vi "PRT1_Vi.vi"() -> ()   [LabVIEW 2020]
uses:
  <vilib>/Analysis/3filter.llb/Filter Passband Type.ctl
  <vilib>/Analysis/3filter.llb/Butterworth Filter (DBL).vi
  <vilib>/Analysis/NI_AALBase.lvlib
  <vilib>/ptbypt/NI_PtbyPt.lvlib
panel:
  out "FLUX_GRAPH":dbl(graph)
  out "VOLUME_GRAPH":dbl(graph)
  out "VOLUME [ L ]":dbl
  out "VOLUME_TANK [L]":dbl(slide) scale=0.0..4.0
  out "UPDATED":bool
  out "Respiratoy Rate [bpm]":dbl format="%#_3g"
  out "RESPIRATORY COUNT":dbl
  out "SYSTEM OK":bool
  out "MEAN ERROR":dbl format="%#_4g"
  out "INSPIRATION":bool
  out "SPIRATION":bool
  out "FILTERED VOLTAGE [V]":dbl
  out "VOLTAGE":dbl[](graph)
  in  "STOP SYSTEM":bool
  out "PRESSURE CHART":dbl(graph)
  out "FLUX [L/m]":dbl format="%#_4g"
  out "SPEED[cm/s]":dbl format="%#_4g"
  out "PRESSURE":dbl format="%#_4g"
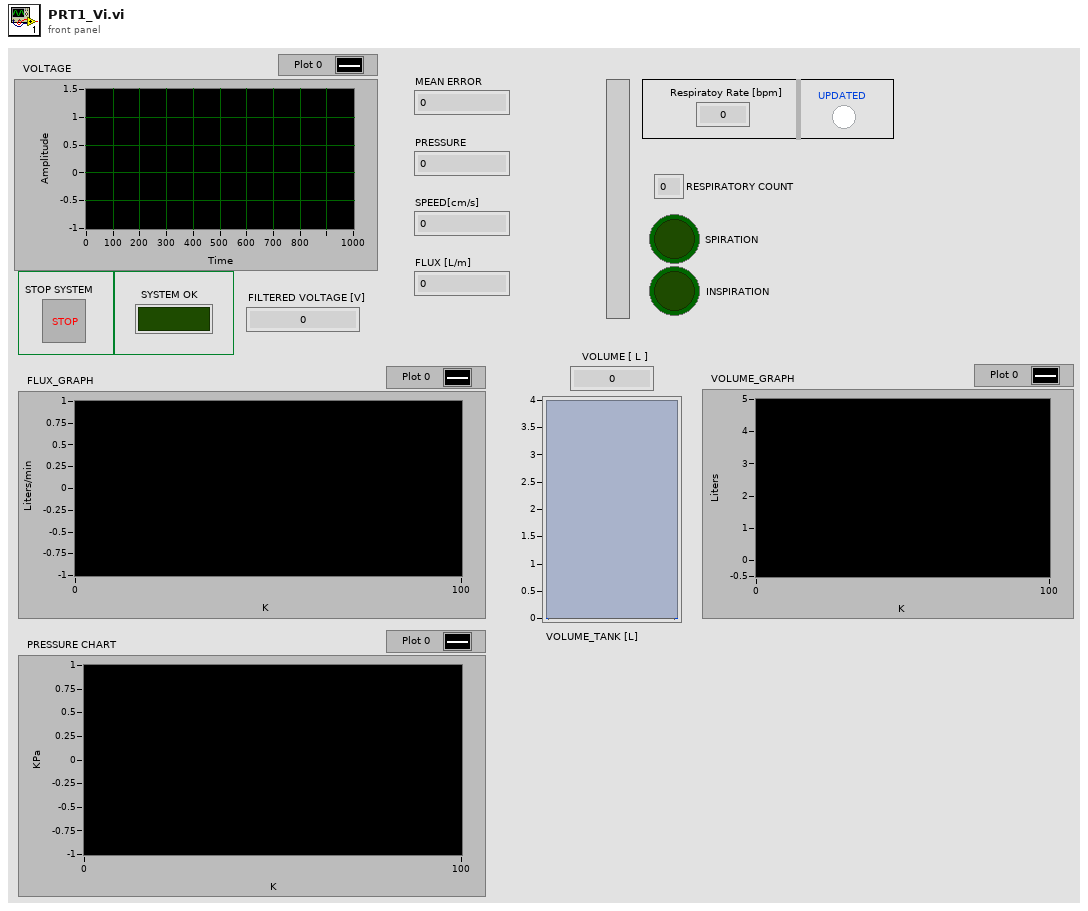
[diagram p1: front panel]
types:
  T1 = typedef "NI_AALBase.lvlib/Filter Passband Type.ctl" = enum32{"Lowpass", "Highpass", "Bandpass", "Bandstop"}
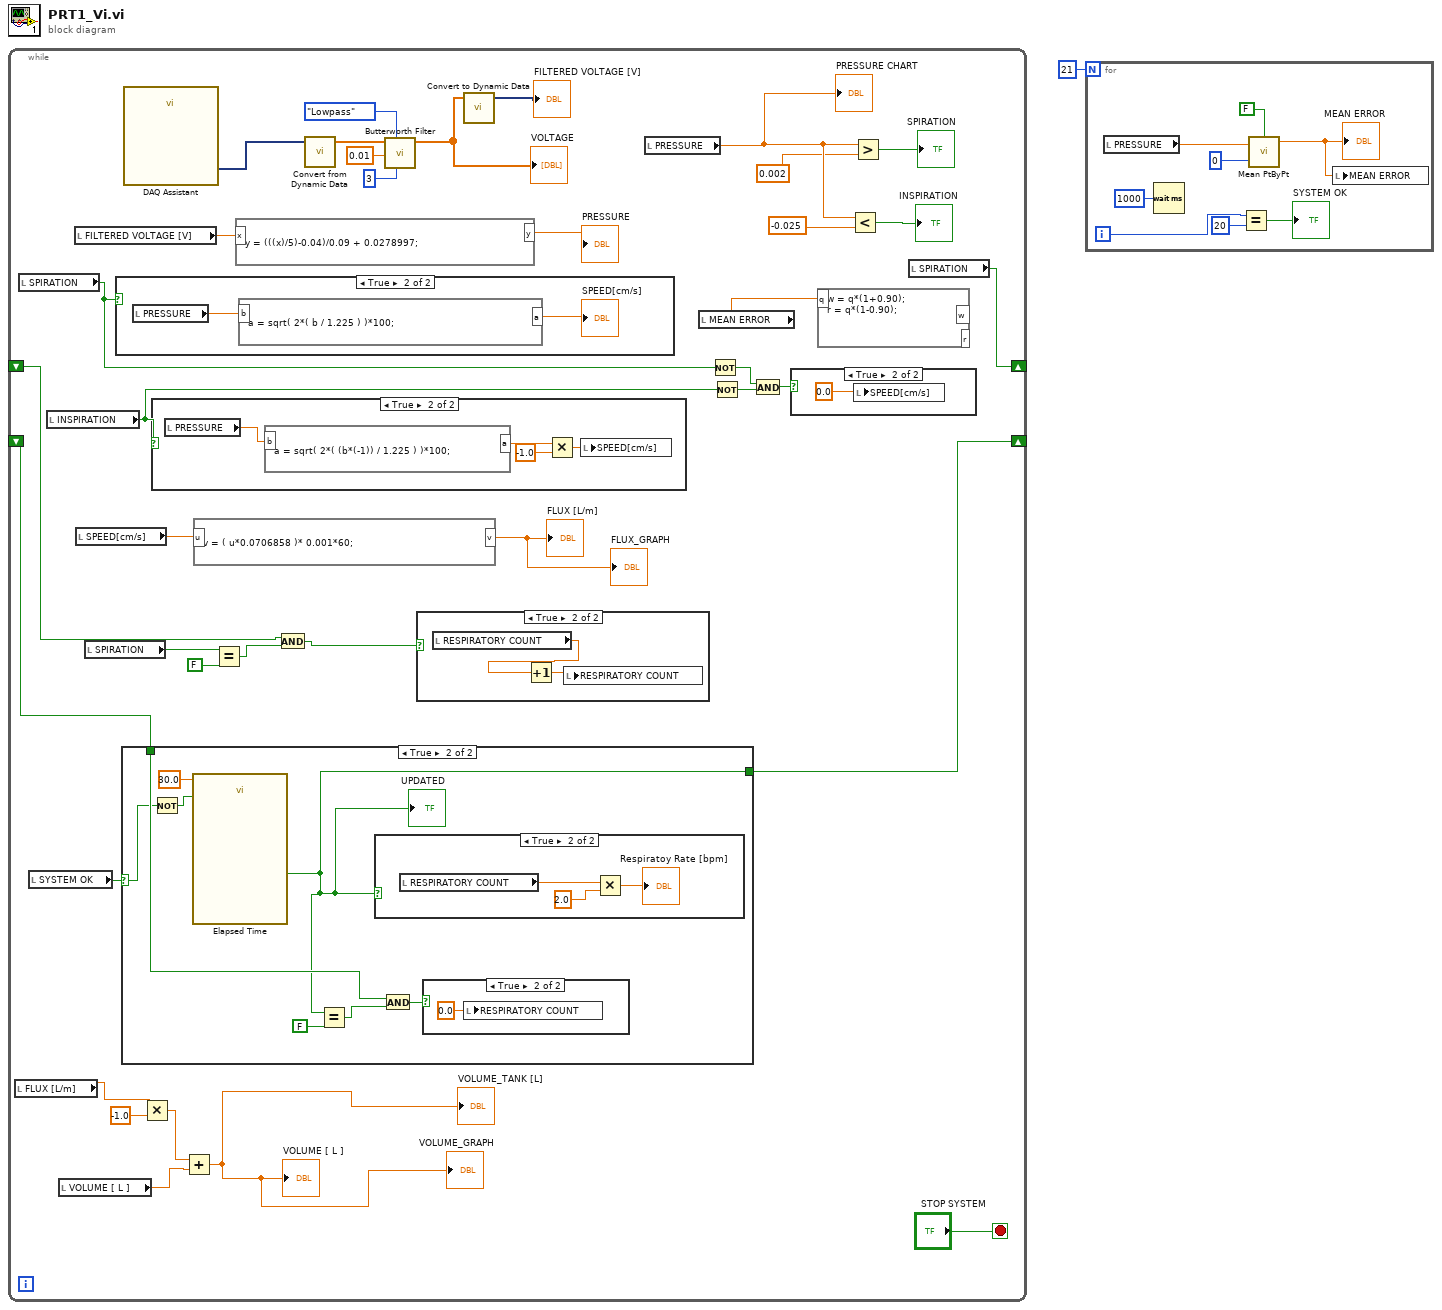
[diagram p0: block diagram]
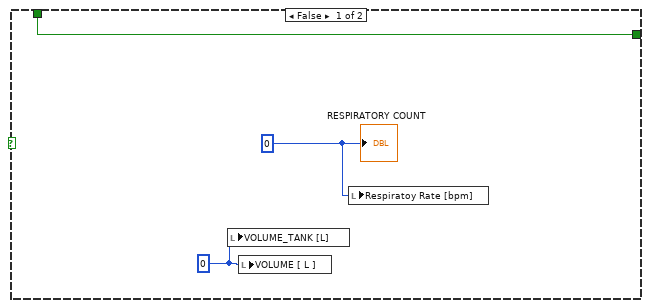
[diagram p5: hidden frame]
diagram:
  n1 = while {
    shift-right: [w25] -> _
    shift-left: _ -> [w24]
    shift-right: [w18] -> _
    shift-left: _ -> [w19]
    stop <- "STOP SYSTEM" stop-if-true
    n2 = local read "FLUX [L/m]"() -> (w3:dbl)
    n3 = local read "SPIRATION"() -> (w9:bool)
    n4 = local read "SYSTEM OK"() -> (w17:bool)
    n5 = local read "INSPIRATION"() -> (w8:bool)
    n6 = local read "VOLUME [ L ]"() -> (w7:dbl)
    n7 = local read "FILTERED VOLTAGE [V]"() -> (w38:dbl)
    n8 = local read "SPEED[cm/s]"() -> (w36:dbl)
    n9 = local read "SPIRATION"() -> (w22:bool)
    n10 = case shown="True" w9 {
      frame False {
      }
      frame True {
        n11 = local read "PRESSURE"() -> (w44:dbl)
        n12 = formula code="a = sqrt( 2*( b / 1.225 ) )*100;"("b"=w44) -> ("a"=→"SPEED[cm/s]":dbl)
      }
    }
    n13 = case shown="True" w17 {
      selector: w17 -> [_ w51]
      tunnel: w19 -> [w47 w53]
      tunnel: [w47 w49] -> w18
      frame False {
        w46 = 0
        w48 = 0
        n14 = local write "VOLUME_TANK [L]"(w46) -> ()
        n15 = local write "VOLUME [ L ]"(w46) -> ()
        n16 = local write "Respiratoy Rate [bpm]"(w48) -> ()
        "RESPIRATORY COUNT" <- w48
      }
      frame True {
        n17 = Not(x=w51) -> (.not. x?=w50:bool)
        n18 = call "Elapsed Time"("Time Target (s)"=30.0, "Reset"=w50) -> ("Time has Elapsed"=w49:bool)  [unwired: 10 in, 7 out]
        "UPDATED" <- w49
        n19 = Equal?(x=w49, y=FALSE) -> (x = y?=w55:bool)
        n20 = case shown="True" w49 {
          frame False {
          }
          frame True {
            n21 = local read "RESPIRATORY COUNT"() -> (w59:dbl)
            n22 = Multiply(x=w59, y=2.0) -> (x*y=→"Respiratoy Rate [bpm]":dbl)
          }
        }
        n23 = And(x=w53, y=w55) -> (x .and. y?=w52:bool)
        n24 = case shown="True" w52 {
          frame False {
          }
          frame True {
            n25 = local write "RESPIRATORY COUNT"(0.0 ("RESPIRATORY COUNT")) -> ()
          }
        }
      }
    }
    n26 = call "DAQ Assistant"() -> ("data"=w27:dynamicdata)  [unwired: 17 in, 2 out]
    n27 = Multiply(x=w3, y=-1.0) -> (x*y=w4:dbl)
    n28 = case shown="True" w8 {
      frame False {
      }
      frame True {
        n29 = local read "PRESSURE"() -> (w43:dbl)
        n30 = formula code="a = sqrt( 2*( (b*(-1)) / 1.225 ) )*100;"("b"=w43) -> ("a"=w42:dbl)
        n31 = Multiply(x=w42, y=-1.0) -> (x*y=w40:dbl)
        n32 = local write "SPEED[cm/s]"(w40) -> ()
      }
    }
    n33 = Add(x=w4, y=w7) -> (x+y=→"VOLUME_TANK [L]" →"VOLUME [ L ]" →"VOLUME_GRAPH":dbl)
    n34 = formula code="v = ( u*0.0706858 )* 0.001*60;"("u"=w36) -> ("v"=→"FLUX [L/m]" →"FLUX_GRAPH":dbl)
    n35 = Equal?(x=w22, y=FALSE) -> (x = y?=w23:bool)
    n36 = formula code="y = (((x)/5)-0.04)/0.09 + 0.0278997;"("x"=w38) -> ("y"=→"PRESSURE":dbl)
    n37 = And(x=w24, y=w23) -> (x .and. y?=w20:bool)
    n38 = call "Convert from Dynamic Data"("Dynamic Data Type"=w27) -> ("Array"=w33:dbl[])  [unwired: 3 in]
    n39 = call-poly <vilib>:"Butterworth Filter.vi"("order"=3, "filter type"=Filter_Passband_Type."Lowpass", "low cutoff freq: fl"=0.01, "X"=w33) -> ("Filtered X"=w31:dbl[])  [unwired: 4 in, 1 out]
    "VOLTAGE" <- w31
    n40 = case shown="True" w20 {
      frame False {
      }
      frame True {
        n41 = local read "RESPIRATORY COUNT"() -> (w62:dbl)
        n42 = Increment(x=w62) -> (x+1=w61:dbl)
        n43 = local write "RESPIRATORY COUNT"(w61) -> ()
      }
    }
    n44 = call "Convert to Dynamic Data"("Waveform"=w31) -> ("Dynamic Data Type"=→"FILTERED VOLTAGE [V]":dynamicdata)  [unwired: 3 in]
    n45 = local read "PRESSURE"() -> (w16:dbl)
    "PRESSURE CHART" <- w16
    n46 = local read "MEAN ERROR"() -> (w15:dbl)
    n47 = Not(x=w9) -> (.not. x?=w11:bool)
    n48 = Not(x=w8) -> (.not. x?=w10:bool)
    n49 = And(x=w11, y=w10) -> (x .and. y?=w12:bool)
    n50 = case shown="True" w12 {
      frame False {
      }
      frame True {
        n51 = local write "SPEED[cm/s]"(0.0 ("SPEED[cm/s]")) -> ()
      }
    }
    n52 = formula code="w = q*(1+0.90);\nr = q*(1-0.90);"("q"=w15) -> ()  [unwired: 2 out]
    n53 = Less?(x=w16, y=-0.025) -> (x < y?=→"INSPIRATION":bool)
    n54 = Greater?(x=w16, y=0.002) -> (0:→"SPIRATION":bool)
    n55 = local read "SPIRATION"() -> (w25:bool)
  }
  n56 = for {
    N: 21 -> [_]
    i -> [w66]
    n57 = local read "PRESSURE"() -> (w69:dbl)
    n58 = Wait (ms)(milliseconds to wait=u32 1000) -> ()  [unwired: 1 out]
    n59 = Equal?(x=w66, y=20) -> (x = y?=→"SYSTEM OK":bool)
    n60 = call <vilib>:"Mean PtByPt.vi"("x"=w69, "sample length"=0, "initialize"=FALSE) -> ("mean"=w63:dbl)  [unwired: 1 in, 1 out]
    "MEAN ERROR" <- w63
    n61 = local write "MEAN ERROR"(w63) -> ()
  }
